vi "MAIN.vi"() -> ()   [LabVIEW 2016]
panel:
  in  "Constructor":bool
  in  "Real exp":bool
  in  "Schedule":bool
  in  "Open Space":bool
  in  "СТОП":bool
  in  "НАука":bool
  in  "Устройство станции":bool
  in  "Общая Инфа":bool
  in  "Доставка":bool
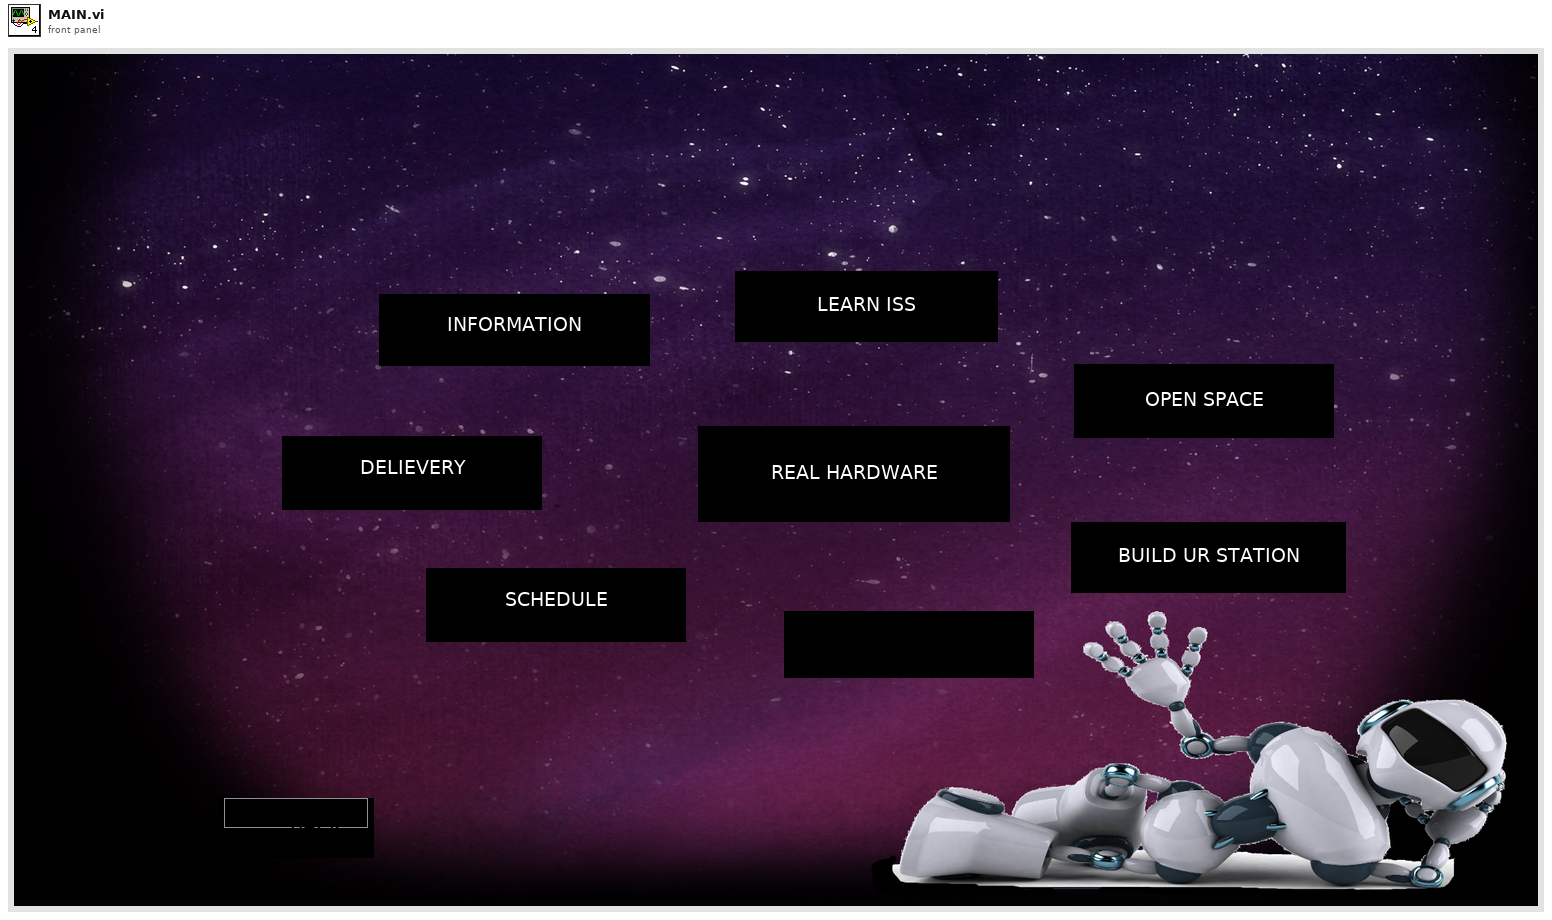
[diagram p1: front panel]
types:
  T1 = enum32{"Invalid", "Standard", "Closed", "Hidden", "Minimized", "Maximized"}
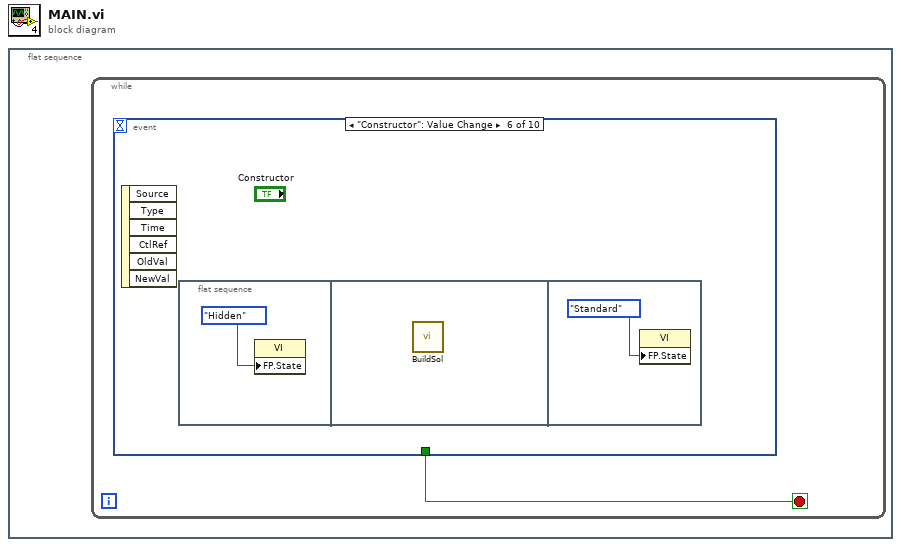
[diagram p0: block diagram]
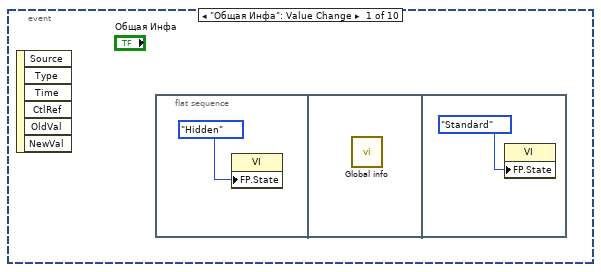
[diagram p2: hidden frame]
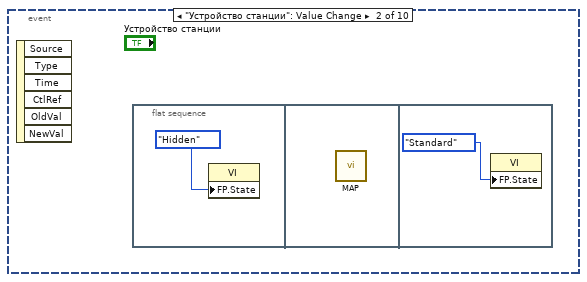
[diagram p3: hidden frame]
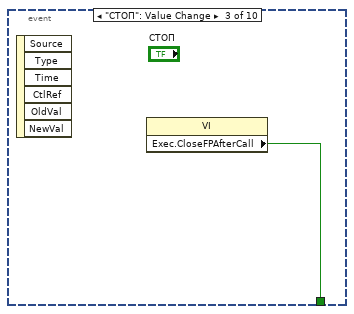
[diagram p4: hidden frame]
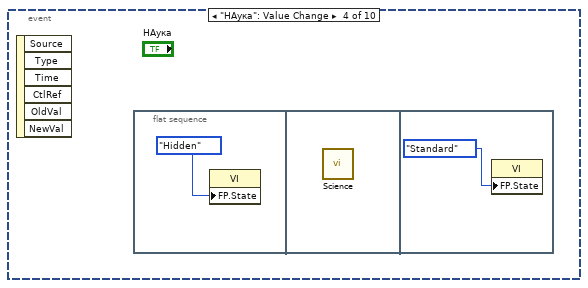
[diagram p5: hidden frame]
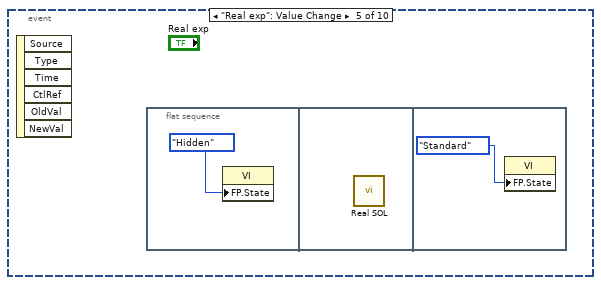
[diagram p6: hidden frame]
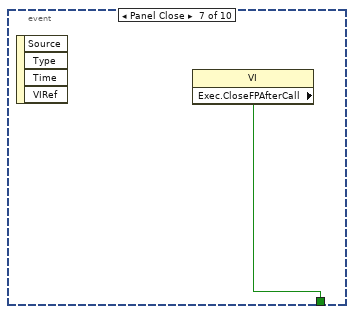
[diagram p7: hidden frame]
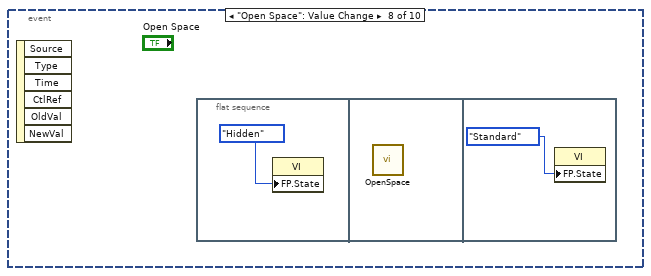
[diagram p8: hidden frame]
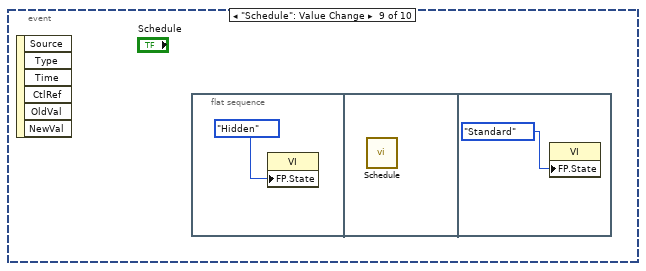
[diagram p9: hidden frame]
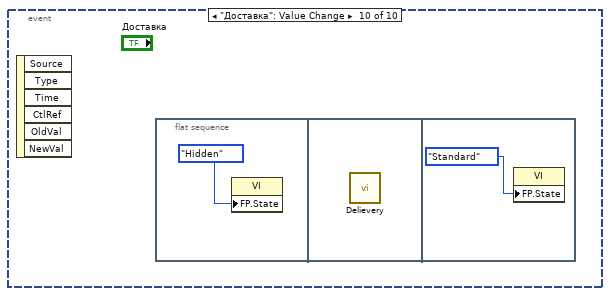
[diagram p10: hidden frame]
diagram:
  n1 = flat-sequence {
    frame #0 {
      n2 = while {
        stop <- w1 stop-if-true
        n3 = event shown="[5] \"Constructor\": Value Change" {
          selector: _ -> [_ _ _ _ _ _ _ _ _ _]
          dyn-events: _ -> [_ _ _ _ _ _ _ _ _ _]
          timeout: _ -> [_ _ _ _ _ _ _ _ _ _]
          tunnel: [_ _ w6 _ _ _ w13 _ _ _] -> w1
          event "Общая Инфа": Value Change {
            n4 = event-data() -> ()  [unwired: 1 in, 6 out]
            n5 = flat-sequence {
              frame #0 {
                n6 = property class="VI"("FP.State"=T1."Hidden" ("Front Panel Window:State")) -> ()  [unwired: 2 in, 2 out]
              }
              frame #1 {
                n7 = call "Global info.vi"() -> ()  [unwired: 12 in]
              }
              frame #2 {
                n8 = property class="VI"("FP.State"=T1."Standard" ("Front Panel Window:State")) -> ()  [unwired: 2 in, 2 out]
              }
            }
          }
          event "Устройство станции": Value Change {
            n9 = event-data() -> ()  [unwired: 1 in, 6 out]
            n10 = flat-sequence {
              frame #0 {
                n11 = property class="VI"("FP.State"=T1."Hidden" ("Front Panel Window:State")) -> ()  [unwired: 2 in, 2 out]
              }
              frame #1 {
                n12 = call "MAP.vi"() -> ()  [unwired: 12 in]
              }
              frame #2 {
                n13 = property class="VI"("FP.State"=T1."Standard" ("Front Panel Window:State")) -> ()  [unwired: 2 in, 2 out]
              }
            }
          }
          event "СТОП": Value Change {
            n14 = event-data() -> ()  [unwired: 1 in, 6 out]
            n15 = property class="VI"() -> ("Exec.CloseFPAfterCall"=w6:bool)  [unwired: 2 in, 2 out]
          }
          event "НАука": Value Change {
            n16 = event-data() -> ()  [unwired: 1 in, 6 out]
            n17 = flat-sequence {
              frame #0 {
                n18 = property class="VI"("FP.State"=T1."Hidden" ("Front Panel Window:State")) -> ()  [unwired: 2 in, 2 out]
              }
              frame #1 {
                n19 = call "Science.vi"() -> ()  [unwired: 12 in]
              }
              frame #2 {
                n20 = property class="VI"("FP.State"=T1."Standard" ("Front Panel Window:State")) -> ()  [unwired: 2 in, 2 out]
              }
            }
          }
          event "Real exp": Value Change {
            n21 = event-data() -> ()  [unwired: 1 in, 6 out]
            n22 = flat-sequence {
              frame #0 {
                n23 = property class="VI"("FP.State"=T1."Hidden" ("Front Panel Window:State")) -> ()  [unwired: 2 in, 2 out]
              }
              frame #1 {
                n24 = call "Real SOL.vi"() -> ()  [unwired: 12 in]
              }
              frame #2 {
                n25 = property class="VI"("FP.State"=T1."Standard" ("Front Panel Window:State")) -> ()  [unwired: 2 in, 2 out]
              }
            }
          }
          event "Constructor": Value Change {
            n26 = event-data() -> ()  [unwired: 1 in, 6 out]
            n27 = flat-sequence {
              frame #0 {
                n28 = property class="VI"("FP.State"=T1."Hidden" ("Front Panel Window:State")) -> ()  [unwired: 2 in, 2 out]
              }
              frame #1 {
                n29 = call "BuildSol.vi"() -> ()  [unwired: 12 in]
              }
              frame #2 {
                n30 = property class="VI"("FP.State"=T1."Standard" ("Front Panel Window:State")) -> ()  [unwired: 2 in, 2 out]
              }
            }
          }
          event Panel Close {
            n31 = event-data() -> ()  [unwired: 1 in, 4 out]
            n32 = property class="VI"() -> ("Exec.CloseFPAfterCall"=w13:bool)  [unwired: 2 in, 2 out]
          }
          event "Open Space": Value Change {
            n33 = event-data() -> ()  [unwired: 1 in, 6 out]
            n34 = flat-sequence {
              frame #0 {
                n35 = property class="VI"("FP.State"=T1."Hidden" ("Front Panel Window:State")) -> ()  [unwired: 2 in, 2 out]
              }
              frame #1 {
                n36 = call "OpenSpace.vi"() -> ()  [unwired: 12 in]
              }
              frame #2 {
                n37 = property class="VI"("FP.State"=T1."Standard" ("Front Panel Window:State")) -> ()  [unwired: 2 in, 2 out]
              }
            }
          }
          event "Schedule": Value Change {
            n38 = event-data() -> ()  [unwired: 1 in, 6 out]
            n39 = flat-sequence {
              frame #0 {
                n40 = property class="VI"("FP.State"=T1."Hidden" ("Front Panel Window:State")) -> ()  [unwired: 2 in, 2 out]
              }
              frame #1 {
                n41 = call "Schedule.vi"() -> ()  [unwired: 12 in]
              }
              frame #2 {
                n42 = property class="VI"("FP.State"=T1."Standard" ("Front Panel Window:State")) -> ()  [unwired: 2 in, 2 out]
              }
            }
          }
          event "Доставка": Value Change {
            n43 = event-data() -> ()  [unwired: 1 in, 6 out]
            n44 = flat-sequence {
              frame #0 {
                n45 = property class="VI"("FP.State"=T1."Hidden" ("Front Panel Window:State")) -> ()  [unwired: 2 in, 2 out]
              }
              frame #1 {
                n46 = call "Delievery.vi"() -> ()  [unwired: 12 in]
              }
              frame #2 {
                n47 = property class="VI"("FP.State"=T1."Standard" ("Front Panel Window:State")) -> ()  [unwired: 2 in, 2 out]
              }
            }
          }
        }
      }
    }
  }
